vi "Lin_Starten.vi"(8 "error in (no error)":errorcluster caption="Fehler (Eingang, kein Fehler)") -> (0 "error out":errorcluster caption="Fehler (Ausgang)")   [LabVIEW 2020, in "Linearisierung v2.lvlib"]
uses:
  Linearisierung v2.lvlib
  Auto Kalibrieren/Aktion FGV Autokal GT.ctl
  Auto Kalibrieren/Auto Kalibrieren.lvlib
panel:
  in  "error in":errorcluster
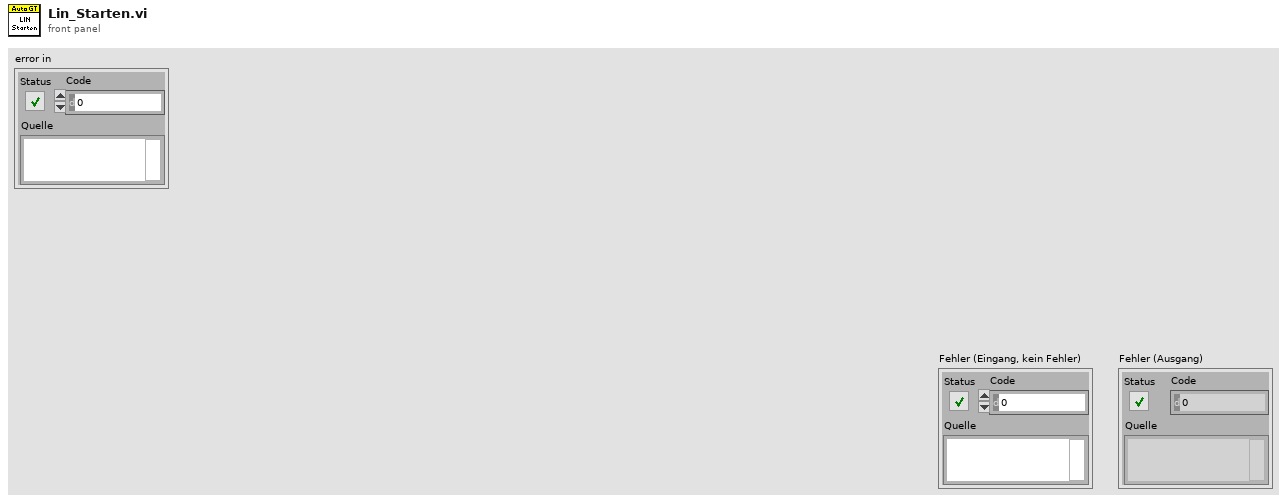
[diagram p1: front panel]
types:
  T1 = typedef "Auto Kalibrieren.lvlib/Aktion FGV Autokal GT.ctl" = enum16{"lesen", "Autokal GT", "Referenz Start"}
  T2 = enum32{"Bad", "Idle", "Run top level", "Running"}
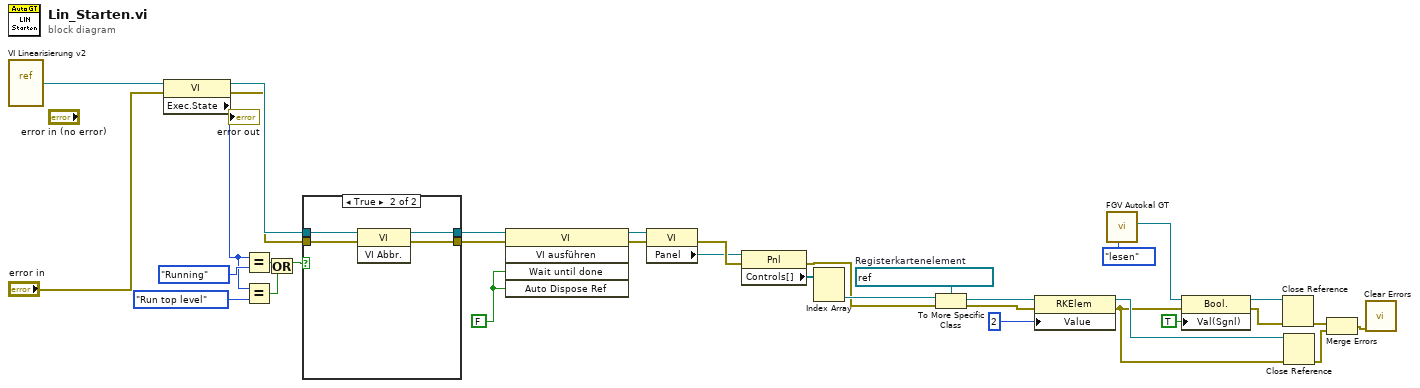
[diagram p0: block diagram]
diagram:
  w20 = refnum<vi> refnum  # Registerkartenelement
  w32 = FALSE
  n1 = vi-ref "VI Linearisierung v2.vi"() -> (w19:refnum<vi>)
  n2 = property class="VI"(reference=w19, error in="error in") -> (reference out=w31:refnum<vi>, error out=w28:errorcluster, "Exec.State"=w25:T2)
  n3 = Equal?(x=w25, y=T2."Running" ("Ausführung:Status")) -> (x = y?=w29:bool)
  n4 = Equal?(x=w25, y=T2."Run top level" ("Ausführung:Status")) -> (x = y?=w24:bool)
  n5 = Or(x=w29, y=w24) -> (x .or. y?=w1:bool)
  n6 = case shown="True" w1 {
    tunnel: w31 -> [w36 w40]
    tunnel: [w36 w39] -> w30
    tunnel: w28 -> [w35 w38]
    tunnel: [w35 w37] -> w27
    frame False {
    }
    frame True {
      n7 = invoke class="VI" method="VI Abbr."(reference=w40, error in=w38) -> (reference out=w39:refnum<vi>, error out=w37:errorcluster)  [unwired: 1 in, 1 out]
    }
  }
  n8 = invoke class="VI" method="VI ausführen"(reference=w30, error in=w27, "Wait until done"=w32, "Auto Dispose Ref"=w32) -> (reference out=w16:refnum<vi>, error out=w15:errorcluster)  [unwired: 1 in, 3 out]
  n9 = property class="VI"(reference=w16, error in=w15) -> (error out=w23:errorcluster, "Panel"=w22:refnum<vi>)  [unwired: 1 out]
  n10 = property class="Pnl"(reference=w22, error in=w23) -> (error out=w13:errorcluster, "Controls[]"=w21:refnum<vi>[])  [unwired: 1 out]
  n11 = Index Array(array=w21) -> (element #2=w17:refnum<vi>)  [unwired: 2 in, 1 out]
  n12 = To More Specific Class(target class=w20, reference=w17, error in=w13) -> (specific class reference=w14:refnum<vi>, error out=w12:errorcluster)
  n13 = property class="RKElem"(reference=w14, error in=w12, "Value"=2) -> (reference out=w6:refnum<vi>, error out=w5:errorcluster)
  n14 = call "FGV Autokal GT.vi"("Aktion FGV AutoKal"=Aktion_FGV_Autokal_GT."lesen") -> ("Start LinCheck"=w10:refnum<vi>)  [unwired: 8 in, 2 out]
  n15 = property class="Bool."(reference=w10, error in=w5, "Val(Sgnl)"=TRUE) -> (reference out=w8:refnum<vi>, error out=w7:errorcluster)
  n16 = Close Reference(reference=w8, error in (no error)=w7) -> (error out=w3:errorcluster)
  n17 = Close Reference(reference=w6, error in (no error)=w5) -> (error out=w2:errorcluster)
  n18 = Merge Errors(w3, w2) -> (w4:errorcluster)
  n19 = call <vilib>:"Clear Errors.vi"("error in (no error)"=w4) -> ()  [unwired: 5 in, 2 out]
